vi "sub_acquisition.vi"(0 "LightField Automation in":refnum<class "LightField Automation.lvclass">, 1 "Acquisition Parameters 2":refnum<vi>[](array[refnum]), 3 "error in (no error)":errorcluster) -> (7 "LightField Automation out":refnum<class "LightField Automation.lvclass">, 8 "CCD":dbl[](array[numeric]), 9 "DAQmx":dbl[][](array[numeric]), 10 "error out":errorcluster)   [LabVIEW 2015]
uses:
  Ligth Field/lightfield-automation-labview/LightField Automation.lvclass
panel:
  out "data":string
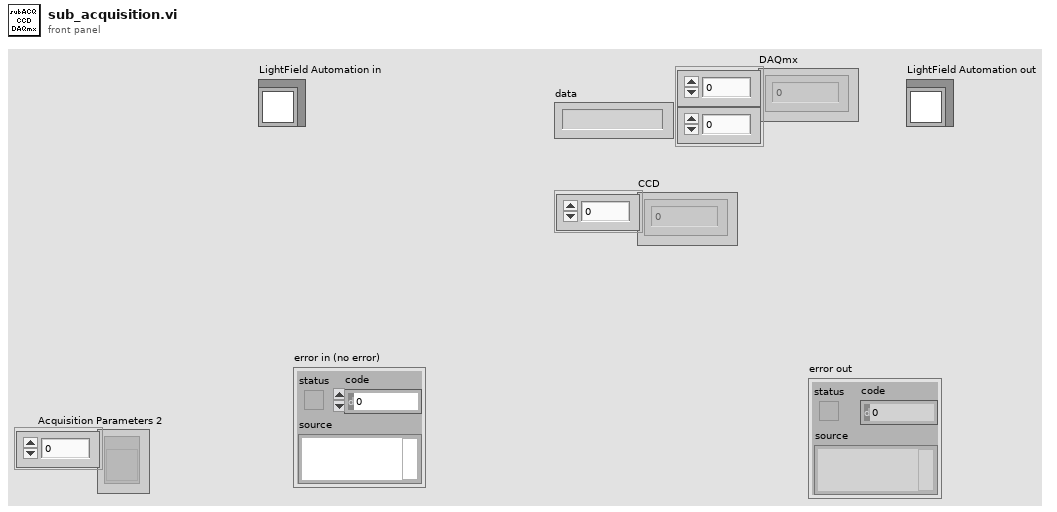
[diagram p1: front panel]
types:
  T1 = cluster{"Image":dbl[][][], "Frame Size":cluster{"F":i32, "Y":i32, "X":i32}}[]
  T2 = cluster{"Image":dbl[][][], "Frame Size":cluster{"F":i32, "Y":i32, "X":i32}}
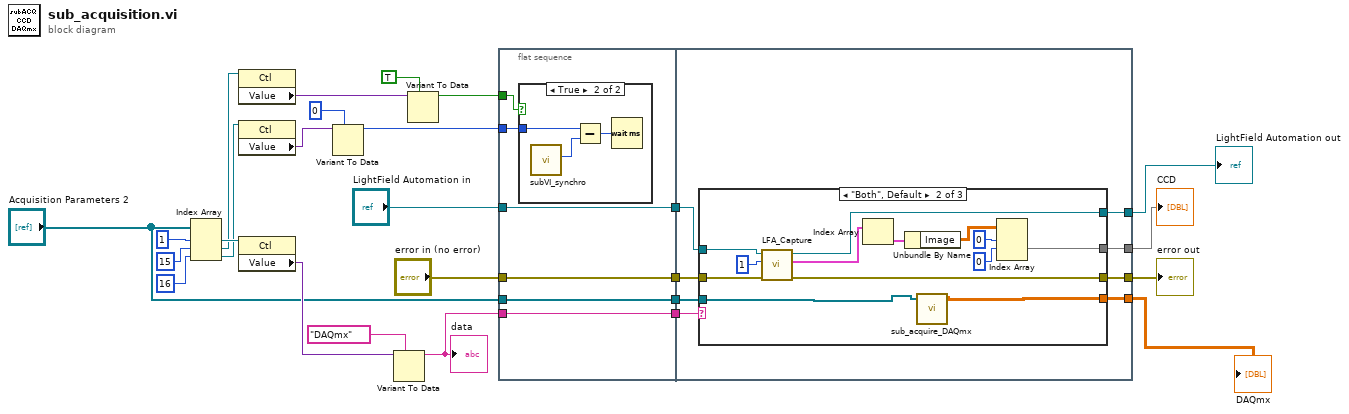
[diagram p0: block diagram]
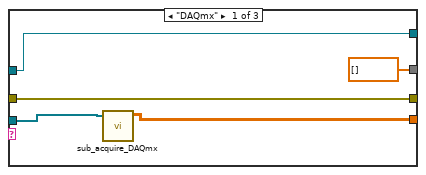
[diagram p3: hidden frame]
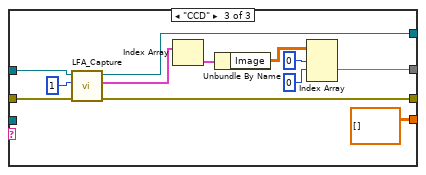
[diagram p4: hidden frame]
diagram:
  n1 = Index Array(array="Acquisition Parameters 2", index #1=1 ("index"), index #2=15 ("index"), index #3=16 ("index")) -> (element #1=w5:refnum<vi>, element #2=w3:refnum<vi>, element #3=w1:refnum<vi>)
  n2 = property on="Property Node" class="Ctl"(reference=w3) -> ("Value"=w16:variant)  [unwired: 1 in, 2 out]
  n3 = property on="Property Node" class="Ctl"(reference=w1) -> ("Value"=w14:variant)  [unwired: 1 in, 2 out]
  n4 = property on="Property Node" class="Ctl"(reference=w5) -> ("Value"=w26:variant)  [unwired: 1 in, 2 out]
  n5 = Variant To Data(type=u32 0, Variant=w14) -> (data=w8:u32)  [unwired: 1 in, 1 out]
  n6 = Variant To Data(type="DAQmx" ("Source"), Variant=w26) -> (data=w17:string)  [unwired: 1 in, 1 out]
  "data" <- w17
  n7 = Variant To Data(type=TRUE, Variant=w16) -> (data=w9:bool)  [unwired: 1 in, 1 out]
  n8 = flat-sequence {
    tunnel: [w32] -> w13
    tunnel: [w31] -> w12
    tunnel: [w30] -> w11
    tunnel: [w29] -> w10
    tunnel: "Acquisition Parameters 2" -> [w32]
    tunnel: "LightField Automation in" -> [w31]
    tunnel: "error in (no error)" -> [w30]
    tunnel: w17 -> [w29]
    tunnel: w9 -> [w28]
    tunnel: w8 -> [w27]
    tunnel: w13 -> [w43]
    tunnel: w12 -> [w40]
    tunnel: w11 -> [w39]
    tunnel: w10 -> [w36]
    tunnel: [w42] -> w23
    tunnel: [w41] -> w22
    tunnel: [w38] -> w19
    tunnel: [w37] -> w18
    frame #0 {
      n9 = case shown="True" w28 {
        tunnel: w27 -> [_ w35]
        frame False {
        }
        frame True {
          n10 = call "subVI_synchro.vi"() -> ("synchro (ms)"=w33:u32)  [unwired: 11 in]
          n11 = Subtract(x=w35, y=w33) -> (x-y=w34:u32)
          n12 = Wait (ms)(milliseconds to wait=w34) -> ()  [unwired: 1 out]
        }
      }
    }
    frame #1 {
      n13 = case shown="\"Both\", Default" w36 {
        tunnel: [dbl[] [] ("array") w52 w66] -> w42
        tunnel: [w45 w49 dbl[][] [] ("data")] -> w41
        tunnel: w43 -> [w44 w50 _]
        tunnel: w40 -> [w47 w56 w70]
        tunnel: w39 -> [w46 w55 w69]
        tunnel: [w47 w53 w68] -> w38
        tunnel: [w46 w54 w67] -> w37
        frame "DAQmx" {
          n14 = call "sub_acquire_DAQmx.vi"("Acquisition Parameters 2"=w44) -> ("data"=w45:dbl[][])  [unwired: 6 in]
        }
        frame "Both", Default {
          n15 = call "LFA_Capture.vi"("error in (no error)"=w55, "Frames"=1, "LightField Automation in"=w56) -> ("error out"=w54:errorcluster, "Data"=w59:T1, "LightField Automation out"=w53:refnum<class "LightField Automation.lvclass">)  [unwired: 6 in]
          n16 = Index Array(array=w59) -> (element=w61:T2)  [unwired: 1 in]
          n17 = Unbundle By Name(w61) -> ("Image"=w60:dbl[][][])
          n18 = call "sub_acquire_DAQmx.vi"("Acquisition Parameters 2"=w50) -> ("data"=w49:dbl[][])  [unwired: 6 in]
          n19 = Index Array(array=w60, index (dim 0)=0 ("index (page)"), index (dim 1)=0 ("disabled index (row)")) -> (element=w52:dbl[])  [unwired: 1 in]
        }
        frame "CCD" {
          n20 = call "LFA_Capture.vi"("error in (no error)"=w69, "Frames"=1, "LightField Automation in"=w70) -> ("error out"=w67:errorcluster, "Data"=w71:T1, "LightField Automation out"=w68:refnum<class "LightField Automation.lvclass">)  [unwired: 6 in]
          n21 = Index Array(array=w71) -> (element=w73:T2)  [unwired: 1 in]
          n22 = Unbundle By Name(w73) -> ("Image"=w72:dbl[][][])
          n23 = Index Array(array=w72, index (dim 0)=0 ("index (page)"), index (dim 1)=0 ("disabled index (row)")) -> (element=w66:dbl[])  [unwired: 1 in]
        }
      }
    }
  }
  "CCD" <- w23
  "error out" <- w18
  "LightField Automation out" <- w19
  "DAQmx" <- w22
